vi "Search Single.vi"(8 "error in (no error)":errorcluster, 10 "Search":string, 11 "all rows":string[][](array[string])) -> (0 "error out":errorcluster, 2 "Array Output":string[](array[string]), 3 "Output":string)   [LabVIEW 2016]
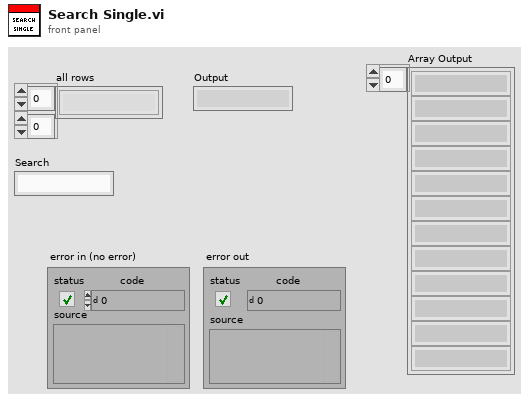
[diagram p1: front panel]
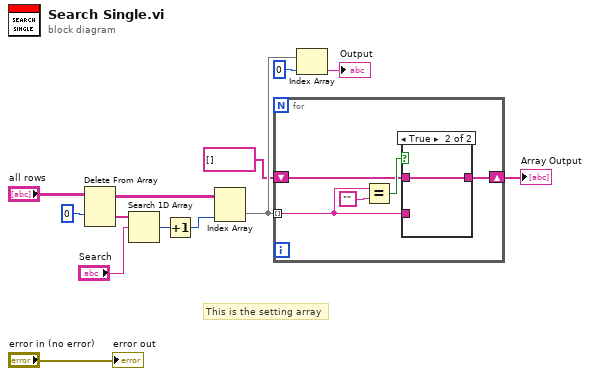
[diagram p0: block diagram]
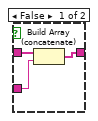
[diagram p2: hidden frame]
diagram:
  # "This is the setting array"
  n1 = Delete From Array(array="all rows", index (row)=0) -> (deleted portion=w6:string[], array with subset deleted=w7:string[][])  [unwired: 2 in]
  n2 = Search 1D Array(1D array=w6, element="Search") -> (index of element=w5:i32)  [unwired: 1 in]
  n3 = Increment(x=w5) -> (x+1=w9:i32)
  n4 = Index Array(array=w7, index (col)=w9) -> (element=w3:string[])  [unwired: 1 in]
  n5 = for {
    tunnel: w3 -> [w14] mode=indexing
    shift-right: [w15] -> w1
    shift-left: string[] [] -> [w16]
    n6 = Equal?(x=w14, y="") -> (x = y?=w17:bool)
    n7 = case shown="True" w17 {
      tunnel: w16 -> [w21 w22]
      tunnel: [w20 w22] -> w15
      tunnel: w14 -> [w19 _]
      frame False {
        n8 = Build Array (concatenate)(w21, w19) -> (w20:string[])
      }
      frame True {
      }
    }
  }
  "Array Output" <- w1
  n9 = Index Array(array=w3, index=0) -> (element=→"Output":string)
  "error out" <- "error in (no error)"
